vi "uStringManipulation_DO.vi"(8 "error in (no error)":errorcluster, 10 "String in":string, 11 "in":refnum<class "1-to-1_map.lvclass">) -> (0 "error out":errorcluster, 2 "String":string, 3 "out":refnum<class "1-to-1_map.lvclass">)   [LabVIEW 2023, in "uLib.lvlib" / "1-to-1_map.lvclass"]
uses:
  1-to-1_map.lvclass
  1-to-1_map.lvclass/1-to-1_map.ctl
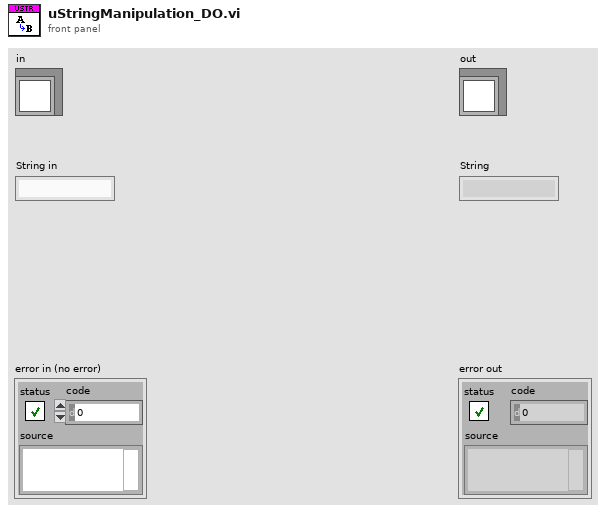
[diagram p1: front panel]
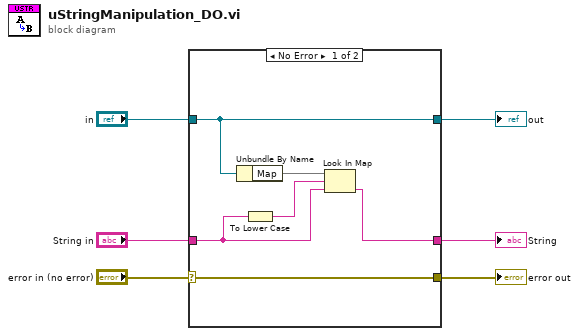
[diagram p0: block diagram]
diagram:
  n1 = case shown="No Error" "error in (no error)" {
    selector: "error in (no error)" -> [w12 w14]
    tunnel: [w12 w14] -> w5
    tunnel: "in" -> [w11 w15]
    tunnel: [w11 w15] -> w3
    tunnel: [w7 w13] -> w2
    tunnel: "String in" -> [w8 w13]
    frame No Error {
      n2 = Unbundle By Name(w11) -> ("Map"=w10:map{string, string})
      n3 = To Lower Case(string=w8) -> (all lower case string=w9:string)
      n4 = Look In Map(map=w10, key=w9, default value=w8) -> (value=w7:string)  [unwired: 1 out]
    }
    frame Error {
    }
  }
  "error out" <- w5
  "out" <- w3
  "String" <- w2
